vi "Open Config File.vi"(8 "error in (no error)":errorcluster, 10 "create file if necessary (T)":bool=TRUE, 11 "Configuration File In":refnum<class "Configuration.lvclass">) -> (0 "error out":errorcluster, 1 "file created?":bool, 3 "Configuration File Out":refnum<class "Configuration.lvclass">)   [LabVIEW 2020, in "Configuration.lvclass"]
doc: "High-level function for opening configuration file data from process class."
uses:
  Configuration.lvclass
  <vilib>/Utility/config.llb/NI_LVConfig.lvlib
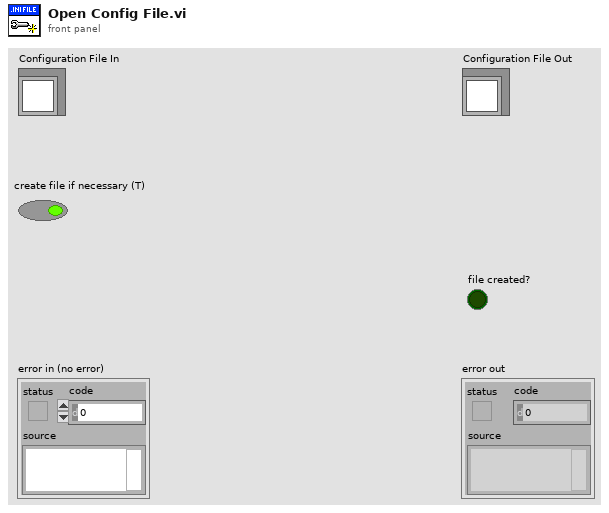
[diagram p1: front panel]
types:
  T1 = typedef "NI_LVConfig.lvlib/Config Data RefNum.ctl" = refnum<k1>
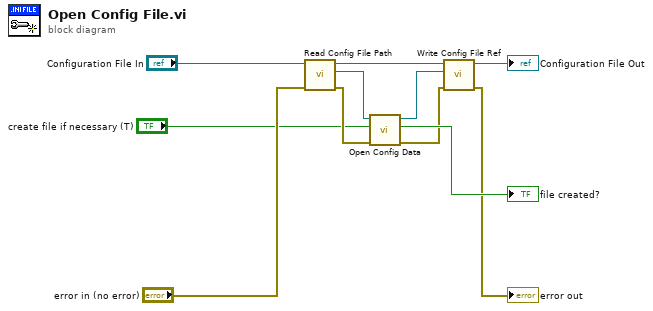
[diagram p0: block diagram]
diagram:
  n1 = call-dynamic "Read Config File Path.vi"("error in (no error)"="error in (no error)", "Configuration File In"="Configuration File In") -> ("error out"=w8:errorcluster, "Config File Path"=w7:path, "Configuration File Out"=w10:refnum<class "Configuration.lvclass">)  [unwired: 7 in]
  n2 = call <vilib>:"Open Config Data.vi"("error in (no error)"=w8, "create file if necessary (T)"="create file if necessary (T)", "configuration file path"=w7) -> ("error out"=w2:errorcluster, "file created?"=→"file created?":bool, "refnum"=w3:T1)  [unwired: 6 in]
  n3 = call-dynamic "Write Config File Ref.vi"("error in (no error)"=w2, "refnum in"=w3, "Configuration File In"=w10) -> ("error out"=→"error out":errorcluster, "Configuration File Out"=→"Configuration File Out":refnum<class "Configuration.lvclass">)  [unwired: 7 in]
